vi "libssh2_knownhost_writefile - invalid known hosts collection - does not return error 1097.vi"() -> ()   [LabVIEW 2013, in "libssh2_tests.lvlib"]
uses:
  libssh2_tests.lvlib
  libssh2/Known Hosts Collection Refnum.ctl
  libssh2/libssh2_init (Default).vi
  <vilib>/addons/_JKI Toolkits/Caraya/classes/Assert/Assert Not Equal Value_Variant.vi
  <vilib>/addons/_JKI Toolkits/Caraya/classes/Test/Test.lvclass
  libssh2/libssh2.lvlib
  <vilib>/addons/_JKI Toolkits/Caraya/classes/Assert/Assert.lvclass
panel:
  out "error out":errorcluster
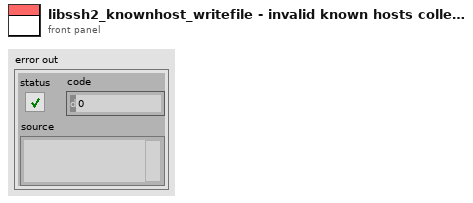
[diagram p1: front panel]
types:
  T1 = typedef "libssh2.lvlib/Known Hosts Collection Refnum.ctl" = refnum<k1>
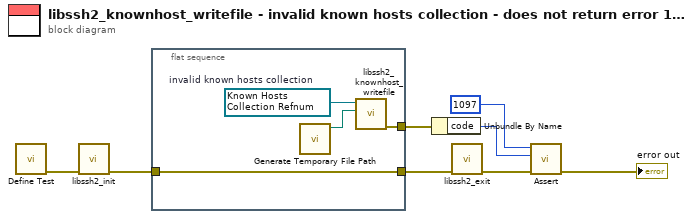
[diagram p0: block diagram]
diagram:
  n1 = call <vilib>:"Define Test.vi"() -> ("error out"=w6:errorcluster)  [unwired: 10 in, 1 out]
  n2 = call-poly "libssh2_init.vi"("error in (no error)"=w6) -> ("error out"=w5:errorcluster)  [unwired: 10 in]
  n3 = flat-sequence {
    tunnel: w5 -> [w12]
    tunnel: [w12] -> w4
    tunnel: [w10] -> w3
    frame #0 {
      w11 = T1 refnum items=["Known Hosts"]  # invalid known hosts collection
      n4 = call <vilib>:"Generate Temporary File Path.vi"() -> ("Unique Temporary File Path"=w9:path)  [unwired: 10 in, 1 out]
      n5 = call "libssh2_knownhost_writefile.vi"("filename"=w9, "known hosts collection"=w11) -> ("error out"=w10:errorcluster)  [unwired: 9 in]
    }
  }
  n6 = Unbundle By Name(w3) -> ("code"=w2:i32)
  n7 = call "libssh2_exit.vi"("error in (no error)"=w4) -> ("error out"=w7:errorcluster)  [unwired: 10 in]
  n8 = call-poly <vilib>:"Assert.vi"("error in (no error)"=w7, "Y"=w2, "X"=1097 ("code")) -> ("error out"=→"error out":errorcluster)  [unwired: 7 in, 1 out]
